vi "calibrationElectrometer_getEvent_IntegrationTime.vi"(8 "error in (no error)":errorcluster, 11 "logevent_IntegrationTime_Ctl":T1) -> (0 "error out":errorcluster, 2 "function return":i32, 3 "logevent_IntegrationTime_Ctl out":T1)   [LabVIEW 2016, in "SALLV_calibrationElectrometer.lvlib"]
doc: "int calibrationElectrometer_shm_getEvent_IntegrationTimeLV(calibrationElectrometer_logevent_IntegrationTimeLV *logevent_IntegrationTime_Ctl );"
uses:
  SALLV_calibrationElectrometer.lvlib
  DataTypes/logevent_IntegrationTime.ctl
  SALLV_calibrationElectrometer.so
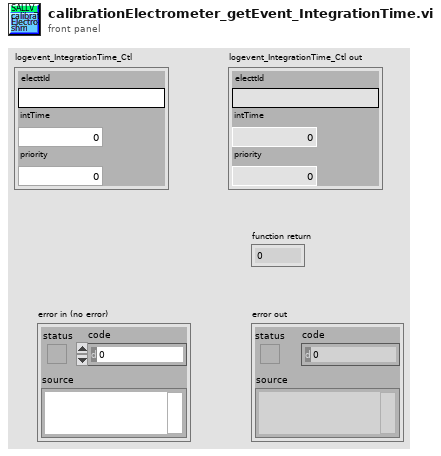
[diagram p1: front panel]
types:
  T1 = typedef "SALLV_calibrationElectrometer.lvlib/logevent_IntegrationTime.ctl" = cluster{"electtId":string, "intTime":sgl, "priority":i32}
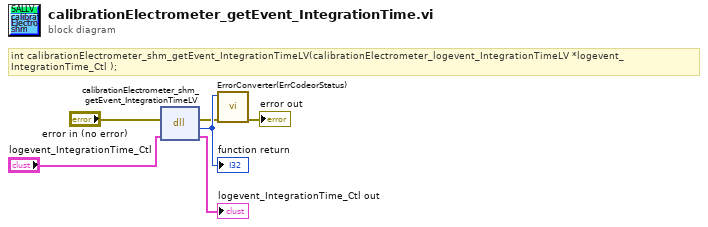
[diagram p0: block diagram]
diagram:
  # "int calibrationElectrometer_shm_getEvent_IntegrationTimeLV(calibrationElectrometer_logevent_IntegrationTimeLV *logevent_IntegrationTime_Ctl );"
  n1 = dll-call lib="home/andres/Desktop/SALLV_calibrationElectrometer/SALLV_calibrationElectrometer.*" fn="calibrationElectrometer_shm_getEvent_IntegrationTimeLV"(error in="error in (no error)", "logevent_IntegrationTime_Ctl"="logevent_IntegrationTime_Ctl") -> (error out=w2:errorcluster, w6:i32, "logevent_IntegrationTime_Ctl"=→"logevent_IntegrationTime_Ctl out":T1)  [unwired: 2 in, 1 out]
  "function return" <- w6
  n2 = call "ErrorConverter(ErrCodeorStatus).vi"("error in (no error)"=w2, "error code"=w6) -> ("error out"=→"error out":errorcluster)  [unwired: 9 in]
